vi "DisplayErrorOnScreen.vi"(8 "error in (no error)":errorcluster) -> ()   [LabVIEW 2019, in "RT_Game.lvlib" / "Engine.lvclass"]
uses:
  Engine.lvclass
  Coordinate.ctl
  <vilib>/FPGAPlugInAG/myRIO-1900/niLvFpga_Open_myRIO-1900.vi
  <vilib>/Utility/error.llb/Error Cluster From Error Code.vi
  <vilib>/rvi/errors/niLvFpgaAdjustHostInterfaceError.vi
  <vilib>/rvi/interface/nirviOpenFPGA/nirviOpenFPGA.xnode
  FPGA_Interface.ctl
  FPGA Bitfiles/myriogameconsole_FPGATarget_Main_ntsPRcBZGxk.lvbitx
  <vilib>/rvi/interface/nirviMethod/nirviMethod.xnode
  <vilib>/FPGAPlugInAG/myRIO-1900/niLvFpga_WriteFifo_myRIO-1900.vi
  <vilib>/rvi/errors/niLvFpgaMergeErrorWithErrorCode.vi
panel:
  out "error out":errorcluster
  out "message":string=" INSTRUCTIONS:\r\rNormal Use:  When using subVIs that incorporate the error in/error out (or error I/O) structure, place this handler where you want to inform the user of an error, typically at the end of the I/O data path, as the last action of the program.  If the error in error? is ERROR, the handler creates a message describing the error and its source.  If the type of dialog = 1 (default), the message is displayed to the user, who can only acknowedge it.  If the type = 2, the user can acknowledge the message or abort execution; aborting a program with active I/O is not recommended.  If the type = 0, no message is displayed; this is used to process the error programmatically, and the error out cluster elements are wired to individual terminals for that reason.  \r\rOther Use:\n\r\nlocal testing.  To test the error code of a subVI or function that does not have the error I/O structure, you can wire its error code and a source string to the local error code and error source inputs.  If error in error? indicates no error and error code is not equal to 0, the local code and source are substituted for the error in values, and error? is set TRUE (ERROR)."
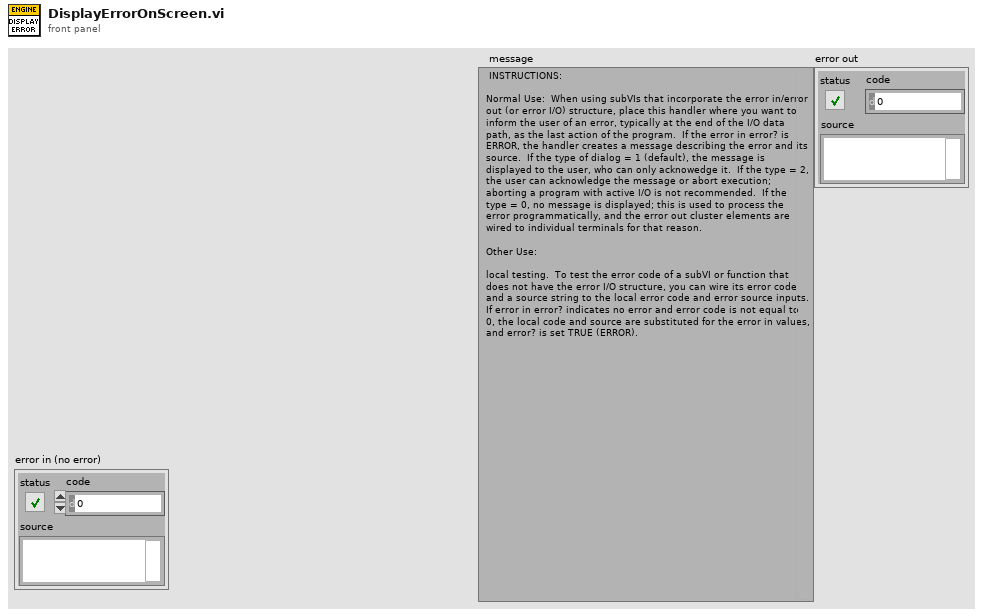
[diagram p1: front panel]
types:
  T1 = typedef "RT_Game.lvlib/Engine.lvclass/Coordinate.ctl" = cluster{"x":dbl, "y":dbl}
  T2 = typedef "FPGA_Interface.ctl" = refnum<k20>
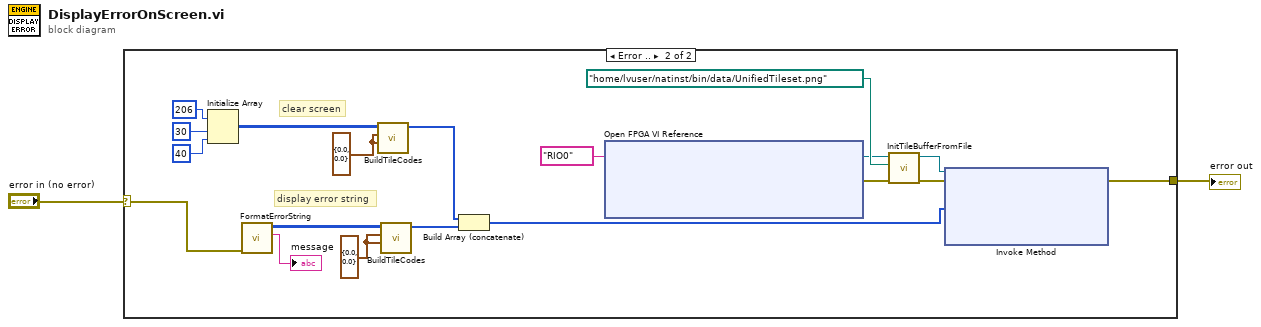
[diagram p0: block diagram]
diagram:
  n1 = case shown="Error .." "error in (no error)" {
    selector: "error in (no error)" -> [w3 w6]
    tunnel: [w3 w4] -> w1
    frame No Error {
    }
    frame Error {
      w15 = T1 {"x"=0.0, "y"=0.0} ("Position")
      w21 = T1 {"x"=0.0, "y"=0.0} ("Position")
      # "display error string"
      # "clear screen"
      n2 = Initialize Array(u32 206, 30 ("dimension size"), 40 ("dimension size")) -> (w16:u32[][])
      n3 = call "FormatErrorString.vi"("error in (no error)"=w6) -> ("message"=→"message":string, "Array"=w20:u32[][])  [unwired: 9 in]
      n4 = call "BuildTileCodes.vi"("CameraPos"=w15, "Position"=w15, "TileCodes"=w16) -> ("Array"=w14:u64[])  [unwired: 8 in]
      n5 = call "BuildTileCodes.vi"("CameraPos"=w21, "Position"=w21, "TileCodes"=w20) -> ("Array"=w12:u64[])  [unwired: 8 in]
      n6 = Build Array (concatenate)(w14, w12) -> (w13:u64[])
      n7 = xnode "Open FPGA VI Reference"("resource name"=tag "RIO0") -> ("FPGA VI Reference Out"=w10:T2, "error out"=w9:errorcluster)  [unwired: 1 in]
      n8 = call "InitTileBufferFromFile.vi"("error in (no error)"=w9, "Tile Path"=path "/home/lvuser/natinst/bin/data/UnifiedTileset.png", "Refnum in"=w10) -> ("error out"=w7:errorcluster, "Refnum out"=w8:T2)  [unwired: 7 in]
      n9 = xnode "Invoke Method"("FPGA VI Reference In"=w8, "error in"=w7, "Data"=w13) -> ("error out"=w4:errorcluster)  [unwired: 1 in, 2 out]
    }
  }
  "error out" <- w1
